vi "FTW-Endpoint-Core-LibraryError.vi"(0 "error in":errorcluster, 7 "Return Value":i64) -> (4 "error out":errorcluster)   [LabVIEW 2013, in "FTW-Actor.lvlib" / "FTW-Endpoint.lvclass"]
uses:
  FTW-Endpoint.lvclass
panel:
  # "Inputs"
  # "Outputs"
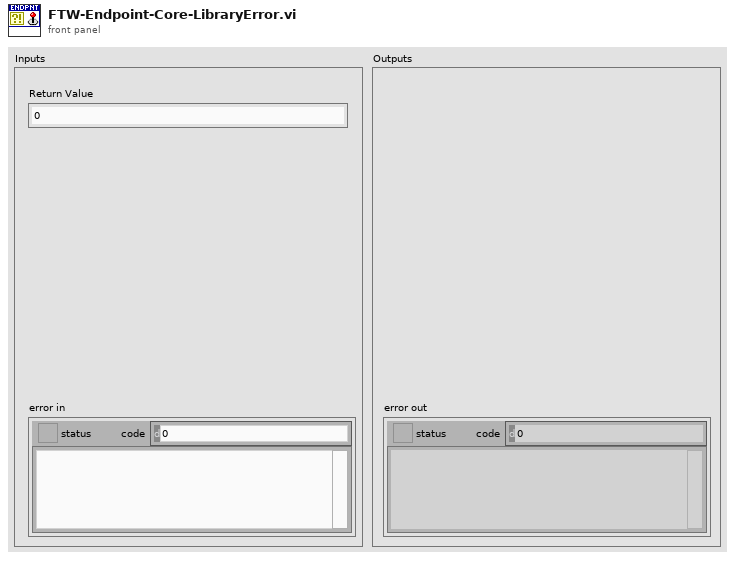
[diagram p1: front panel]
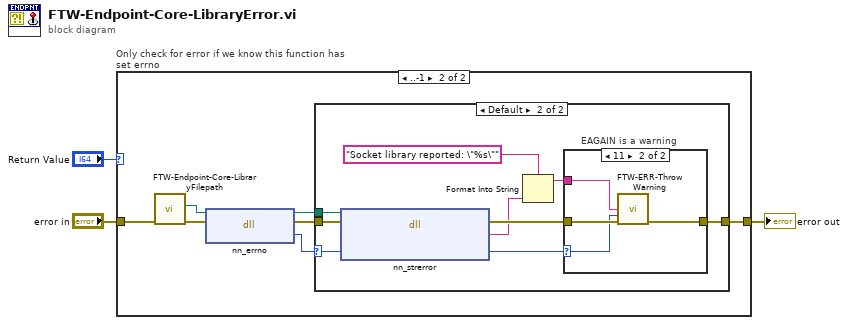
[diagram p0: block diagram]
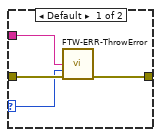
[diagram p4: hidden frame]
diagram:
  n1 = case "Only check for error if we know this function has set errno" shown="..-1" "Return Value" {
    tunnel: [w4 w11] -> w3
    tunnel: "error in" -> [w4 w7]
    frame 0.. {
    }
    frame ..-1 {
      n2 = call "FTW-Endpoint-Core-LibraryFilepath.vi"("error in"=w7) -> ("error out"=w6:errorcluster, "Library Filepath"=w5:path)  [unwired: 8 in, 1 out]
      n3 = dll-call lib="?" fn="nn_errno"(path in=w5, error in=w6) -> (path out=w10:path, error out=w9:errorcluster, "Error Code"=w8:i32)  [unwired: 1 in]
      n4 = case shown="Default" w8 {
        selector: w8 -> [_ w17]
        tunnel: w9 -> [w12 w15]
        tunnel: [w12 w20] -> w11
        tunnel: w10 -> [_ w14]
        frame 0 {
        }
        frame Default {
          n5 = dll-call lib="?" fn="nn_strerror" ("zmq_labview.dll:lvzmq_strerror")(path in=w14, error in=w15, "Error Code from nanomsg"=w17) -> (error out=w21:errorcluster, "Error Description"=w16:string, "Error Code from nanomsg"=w13:i32)  [unwired: 1 in, 1 out]
          n6 = Format Into String(format string="Socket library reported: \"%s\"" ("Error Message"), w16) -> (resulting string=w18:string)  [unwired: 2 in, 1 out]
          n7 = case "EAGAIN is a warning" shown="11" w13 {
            selector: w13 -> [w22 w26]
            tunnel: w21 -> [w25 w29]
            tunnel: [w24 w28] -> w20
            tunnel: w18 -> [w23 w27]
            frame Default {
              n8 = call "FTW-ERR-ThrowError.vi"("Error Message"=w23, "Error Code"=w22, "error in"=w25) -> ("error out"=w24:errorcluster)  [unwired: 12 in]
            }
            frame 11 {
              n9 = call "FTW-ERR-ThrowWarning.vi"("Warning Message"=w27, "Error Code"=w26, "error in"=w29) -> ("error out"=w28:errorcluster)  [unwired: 12 in]
            }
          }
        }
      }
    }
  }
  "error out" <- w3
